vi "kSACommLVClient.vi"(1 "IP Address":string="localhost") -> ()   [LabVIEW 2019]
uses:
  C:/Users/tim/Documents/kSAComm LabView Sample/kSACommInterface.dll
  kSACommInterface.dll
  <vilib>/Platform/TimedLoop/XDataNode/timing_clust.ctl
  <vilib>/Platform/TimedLoop/XDataNode/nitl_modes.ctl
  <vilib>/Platform/TimedLoop/XDataNode/wakeup.ctl
  <vilib>/platform/TimedLoop/XDataNode/XDataNode.xnode
  <vilib>/regexp/Match Regular Expression.xnode
  <vilib>/Platform/TimedLoop/XDataNode/XDNodeRunTimeDep.lvlib
panel:
  out "Laser Command Response":string
  out "Register Data Items":bool
  in  "Laser On/Off":bool
  out "Connected":bool
  out "Exit App":bool
  out "Issue Text Command":bool
  in  "Tab Control":T1(tab)
  in  "Start/Stop Acquire":bool
  in  "Duration Type":i32(ring) items=["DURATION_TIME", "DURATION_DATA_POINTS", "DURATION_UNLIMITED"]
  in  "Run Name":string="LabVIEWTest"
  in  "Number of Samples":i16=1
  in  "Duration":dbl=60.0
  out "Array":cluster{"Id":u32, "Name":string}[](array[cluster])
  out "size(s)":i32
  out "Available Markers":u32
  in  "Show All Markers":bool
  in  "Marker":u32=1
  in  "Table Control":string[][](table)=[["0", "2", "Elapsed Time", " "], ["8", "0", "Data Point", ""], ["41059", "6", "Temperature", ""], ["41029", "6", "Curvature", ""]]
  in  "Data Frequency (ms)":i32=100 min=100 step=100
  out "Text Command Results":string
  in  "Send Text Command":bool
  in  "Command":string(combo)
  out "IssueCommand":i32(ring) items=["ERR_SUCCESS"=0, "ERR_CONNECTION"=-5, "ERR_STATE"=-4, "ERR_PARAM"=-3, "ERR_UNKOWN"=-2, "ERR_GENERAL"=-1]
  out "Last Error":string
  in  "OK Button":bool
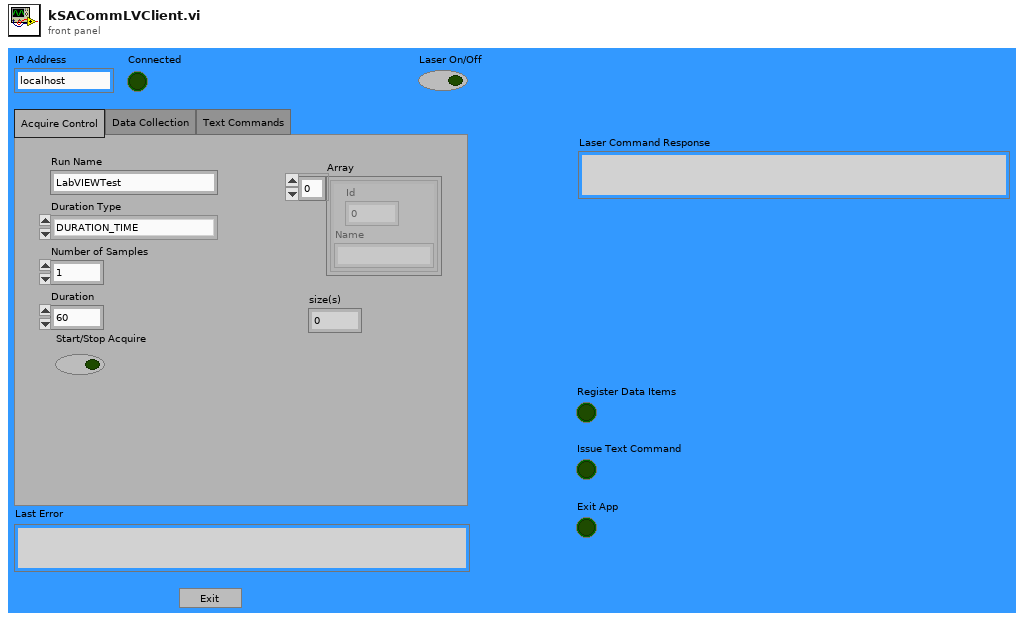
[diagram p1: front panel]
types:
  T1 = enum32{"Acquire Control", "Data Collection", "Text Commands"}
  T2 = typedef "XDNodeRunTimeDep.lvlib/timing_clust.ctl" = cluster{"Expected End [f-1]":u64, "Actual End [f-1]":u64, "Finished Late? [f-1]":bool, "Expected End [i-1]":u64, "Actual End [i-1]":u64, "Finished Late? [i-1]":bool, "Expected Start [i]":u64, "Actual Start [i]":u64, "Expected Start [f]":u64, "Actual Start [f]":u64, "Source Name":string, "Structure Name":string, "Period":i64, "Deadline":i64, "Offset":i64, "Start":i64, "Priority":i32, "Timeout":i32, "Mode":T3, "Wakeup Reason":T4, "Error":errorcluster, "Source Type":string, "Secondary Source Type":string, "Global End Time":u64, "Global Start Time":u64, "Frame Duration":u64, "Iteration Duration":u64, "Assigned CPU":i32, "I/O Scan Engine Mode":u32}
  T3 = typedef "XDNodeRunTimeDep.lvlib/nitl_modes.ctl" = enum32{"No Change", "Process missed periods, maintain original phase", "Discard missed periods, maintain original phase", "Process missed periods, ignore original phase", "Discard missed periods, ignore original phase"}
  T4 = typedef "XDNodeRunTimeDep.lvlib/wakeup.ctl" = enum32{"Normal", "Aborted", "Asynchronous wakeup", "Timing source error", "Timed loop error", "Timeout"}
  T5 = enum8{"Enabled", "Disabled", "Disabled and Grayed Out"}
  T6 = typedef "eventvkey.ctl" = enum16{"ASCII", "Enter", "Return", "Shift", "Ctrl", "Alt", "Cmd", "Opt", "Caps", "NumLock", "Clear", "Break", "Up", "Down", "Left", "Right", "Insert", "Delete", "Home", "End", "PageUp", "PageDown", "Escape", "Help", "Pause", "ScrollLock", "F1", "F2", "F3", "F4", "F5", "F6", "F7", "F8", "F9", "F10", "F11", "F12", "F13", "F14", "F15", "F16", "F17", "F18", "F19", "F20", "F21", "F22", "F23", "F24", "Play", "VolumeUp", "VolumeDown", "Mute", "Two Byte Char"}
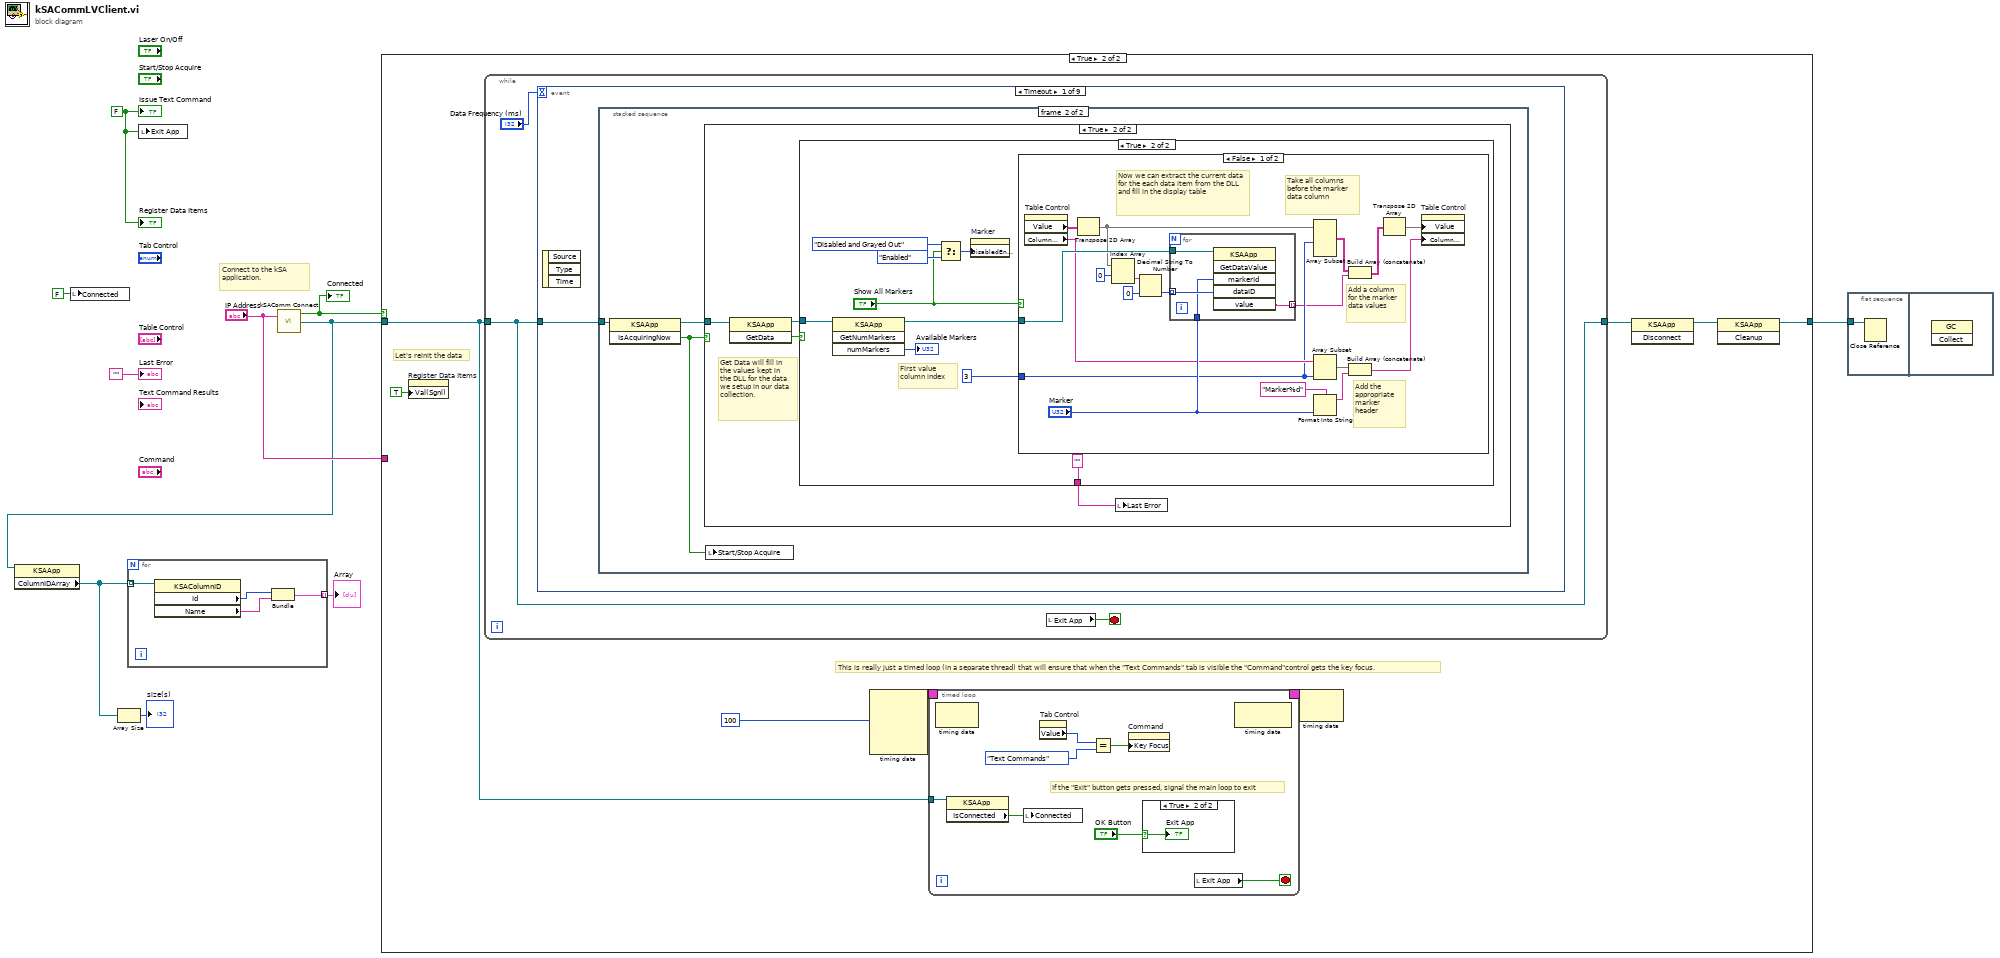
[diagram p0: block diagram]
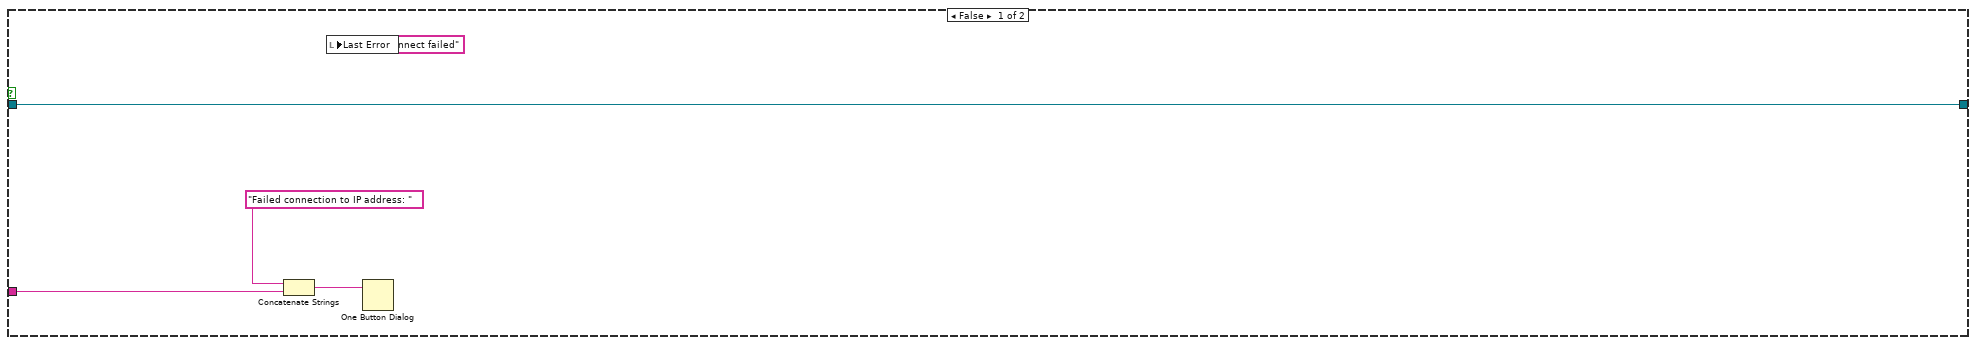
[diagram p2: hidden frame]
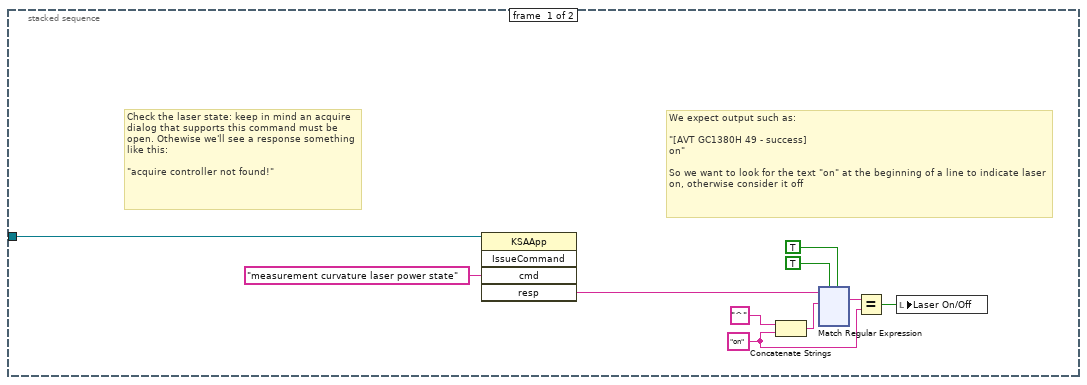
[diagram p4: hidden frame]
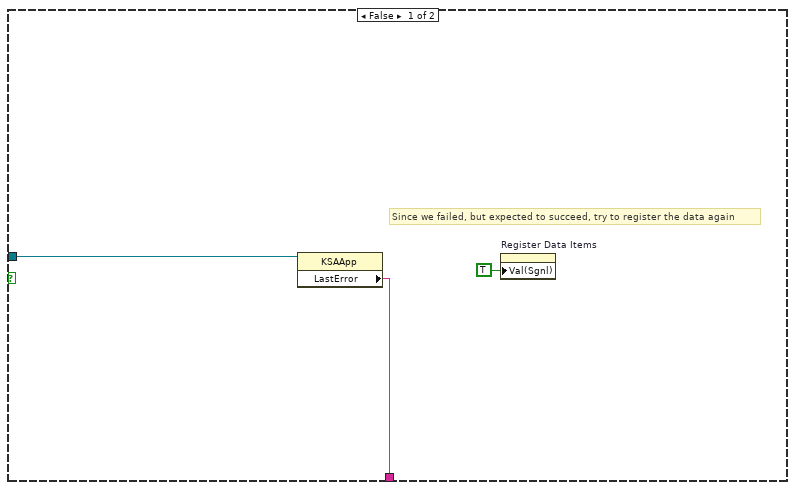
[diagram p6: hidden frame]
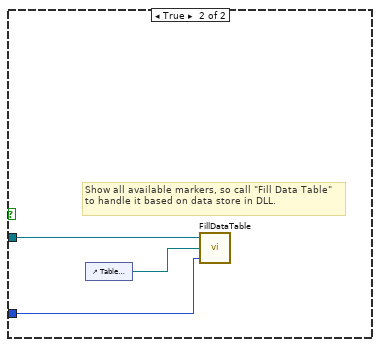
[diagram p7: hidden frame]
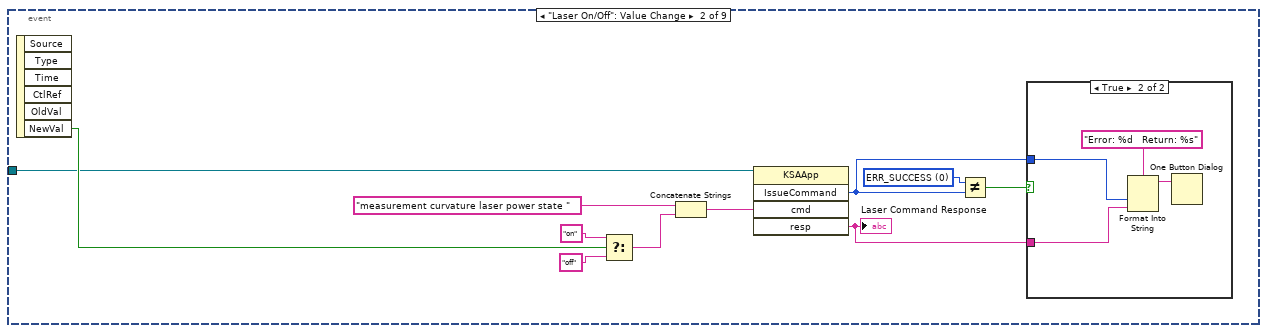
[diagram p8: hidden frame]
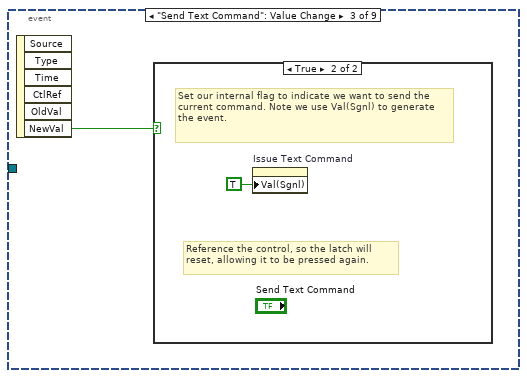
[diagram p10: hidden frame]
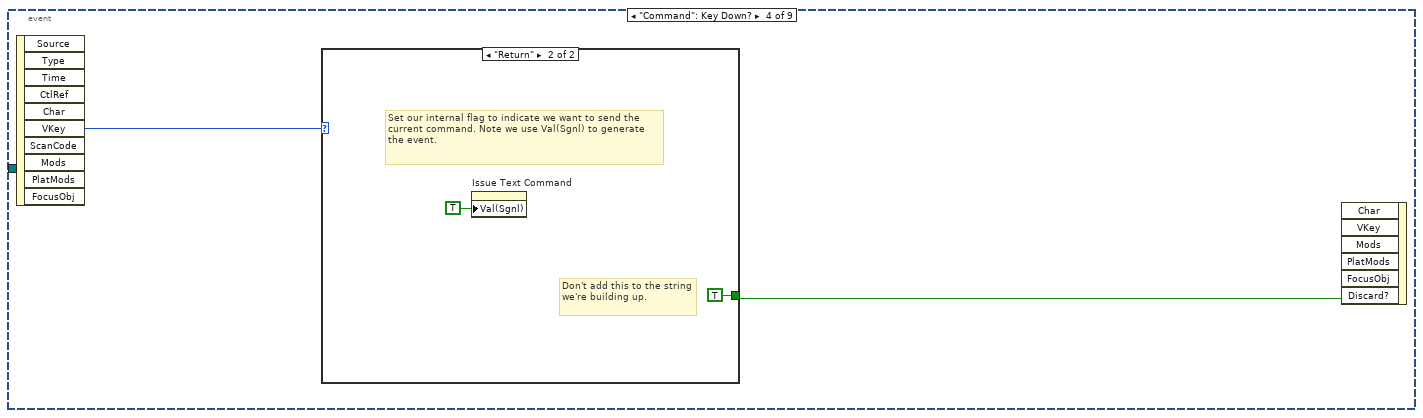
[diagram p12: hidden frame]
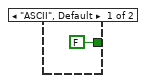
[diagram p13: hidden frame]
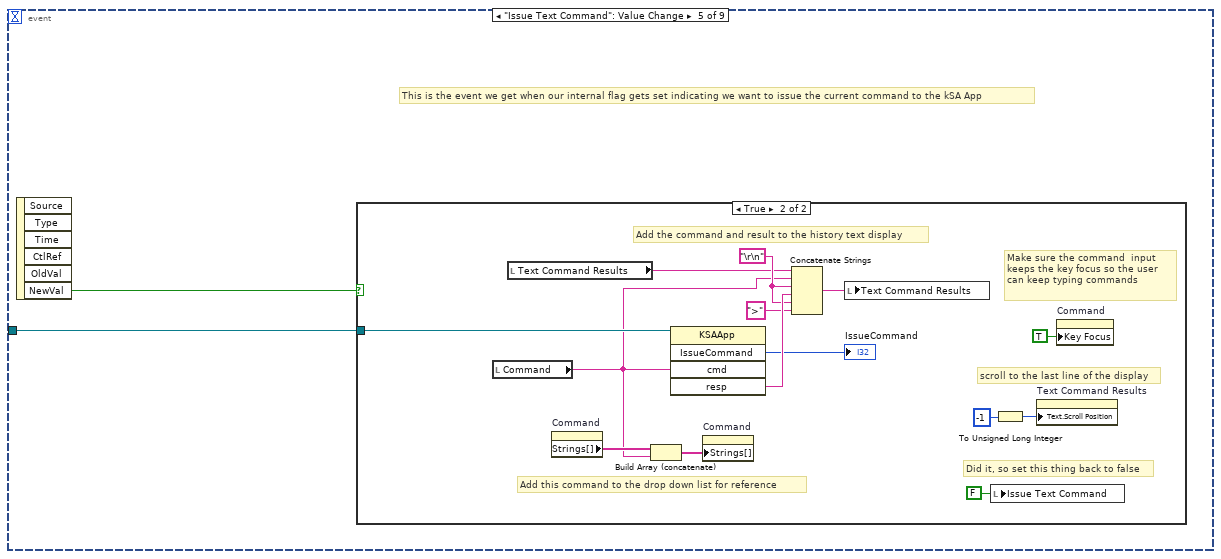
[diagram p14: hidden frame]
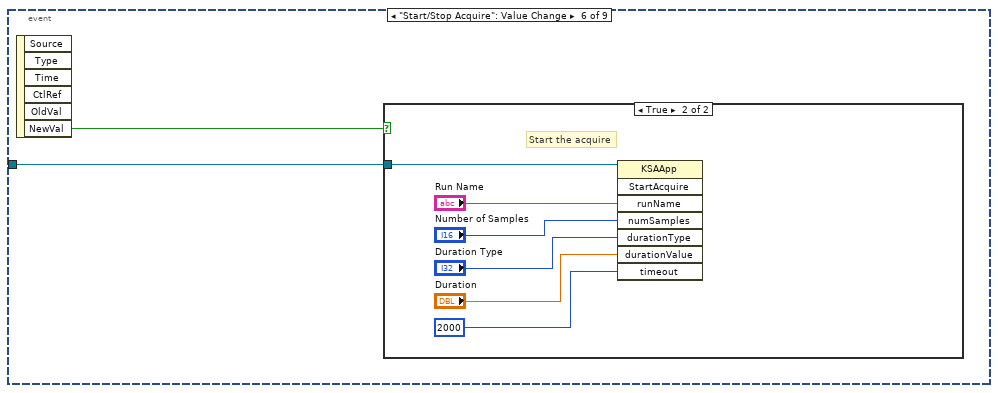
[diagram p16: hidden frame]
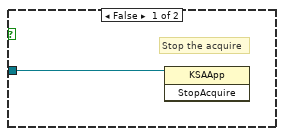
[diagram p17: hidden frame]
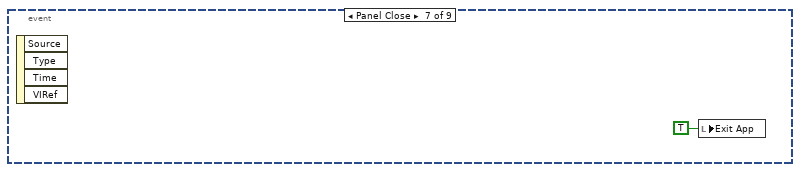
[diagram p18: hidden frame]
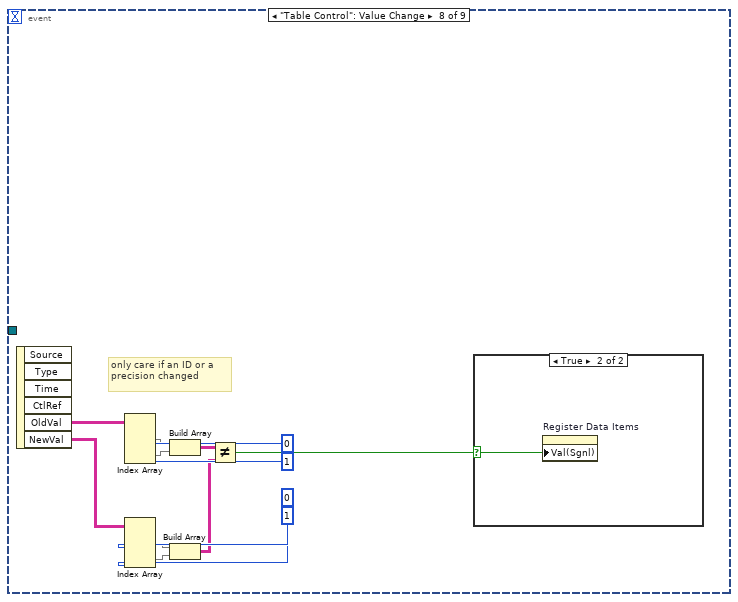
[diagram p19: hidden frame]
diagram:
  w8 = FALSE ("Send Text Command")
  # "Connect to the kSA application."
  n1 = local write "Connected"(FALSE ("Connected")) -> ()
  n2 = local write "Exit App"(w8) -> ()
  n3 = call "kSAComm Connect.vi"("IP Address"="IP Address") -> ("Connect"=w9:bool, "kSAComm ref out"=w4:refnum<k24>)  [unwired: 2 in]
  "Connected" <- w9
  n4 = property class="KSAApp"(reference=w4) -> ("ColumnIDArray"=w2:refnum<k24>[])  [unwired: 1 in, 2 out]
  n5 = Array Size(array=w2) -> (size(s)=→"size(s)":i32)
  n6 = for {
    tunnel: w2 -> [w14] mode=indexing
    tunnel: [w11] -> w3 mode=indexing
    n7 = property class="KSAColumnID"(reference=w14) -> ("Id"=w13:u32, "Name"=w12:string)  [unwired: 1 in, 2 out]
    n8 = Bundle("Id"=w13, "Name"=w12) -> (w11:cluster{"Id":u32, "Name":string})  [unwired: 1 in]
  }
  "Array" <- w3
  n9 = case shown="True" w9 {
    tunnel: w4 -> [w18 w23]
    tunnel: [w18 w21] -> w5
    tunnel: "IP Address" -> [w16 _]
    frame False {
      n10 = Concatenate Strings("Failed connection to IP address: ", w16) -> (w15:string)
      n11 = local write "Last Error"("Connect failed" ("Error")) -> ()
      n12 = One Button Dialog(message=w15) -> ()  [unwired: 1 in, 1 out]
    }
    frame True {
      # "This is really just a timed loop (in a separate thread) that will ensure that when the \"Text Commands\" tab is visible the \"Command\"control gets the key focus."
      # "Let's reinit the data"
      n13 = property on="Register Data Items" class="Bool (strict)"("Val(Sgnl)"=TRUE ("Value (Signaling)")) -> ()  [unwired: 2 in, 2 out]
      n14 = while {
        tunnel: w23 -> [w42]
        tunnel: [w42] -> w20
        stop <- w43 stop-if-true
        n15 = event shown="[0] Timeout" {
          selector: _ -> [_ _ _ _ _ _ _ _ _]
          dyn-events: _ -> [_ _ _ _ _ _ _ _ _]
          timeout: "Data Frequency (ms)" -> [_ _ _ _ _ _ _ _ _]
          tunnel: w42 -> [w45 w215 _ _ w236 w252 _ w263 w278]
          tunnel: [_ _ _ _ _ _ _ w263 _] -> _
          event Timeout {
            n16 = event-data() -> ()  [unwired: 1 in, 3 out]
            n17 = stacked-sequence {
              tunnel: w45 -> [w49 w170]
              frame #0 {
                w46 = "on" ("regular expression")
                # "Check the laser state: keep in mind an acquire dialog that supports this command must be open. Othewise we'll see a response something like this:\n\n\"acquire controller not found!\""
                # "We expect output such as:\n\n\"[AVT GC1380H 49 - success]\non\"\n\nSo we want to look for the text \"on\" at the beginning of a line to indicate laser on, otherwise consider it off"
                n18 = invoke class="KSAApp" method="IssueCommand"(reference=w49, "cmd"="measurement curvature laser power state") -> ("resp"=w55:string)  [unwired: 3 in, 4 out]
                n19 = Concatenate Strings("^", w46) -> (w47:string)
                n20 = xnode "Match Regular Expression"("input string"=w55, "regular expression"=w47, "ignore case? (F)"=TRUE, "multiline? (F)"=TRUE) -> ("whole match"=w52:string)  [unwired: 2 in, 4 out]
                n21 = Equal?(x=w52, y=w46) -> (x = y?=w50:bool)
                n22 = local write "Laser On/Off"(w50) -> ()
              }
              frame #1 {
                n23 = invoke class="KSAApp" method="IsAcquiringNow"(reference=w170) -> (reference out=w172:refnum<k24>, "IsAcquiringNow"=w171:bool)  [unwired: 2 in, 1 out]
                n24 = case shown="True" w171 {
                  tunnel: w172 -> [_ w176]
                  frame False {
                  }
                  frame True {
                    # "Get Data will fill in the values kept in the DLL for the data we setup in our data collection."
                    n25 = invoke class="KSAApp" method="GetData"(reference=w176) -> (reference out=w174:refnum<k24>, "GetData"=w175:bool)  [unwired: 2 in, 1 out]
                    n26 = case shown="True" w175 {
                      tunnel: w174 -> [w179 w181]
                      tunnel: [w178 "" ("LastError")] -> w173
                      frame False {
                        # "Since we failed, but expected to succeed, try to register the data again"
                        n27 = property class="KSAApp"(reference=w179) -> ("LastError"=w178:string)  [unwired: 1 in, 2 out]
                        n28 = property on="Register Data Items" class="Bool (strict)"("Val(Sgnl)"=TRUE ("Value (Signaling)")) -> ()  [unwired: 2 in, 2 out]
                      }
                      frame True {
                        # "First value column index"
                        n29 = invoke class="KSAApp" method="GetNumMarkers"(reference=w181) -> (reference out=w180:refnum<k24>, "numMarkers"=→"Available Markers":u32)  [unwired: 3 in, 2 out]
                        n30 = Select(t=T5."Disabled and Grayed Out" ("Disabled"), s="Show All Markers", f=T5."Enabled" ("Disabled")) -> (s? t:f=w186:T5)
                        n31 = property on="Marker" class="DigNum (strict)"("DisabledEnum"=w186) -> ()  [unwired: 2 in, 2 out]
                        n32 = case shown="False" "Show All Markers" {
                          tunnel: w180 -> [w206 w212]
                          tunnel: 3 ("First Data Column") -> [w193 w211]
                          frame False {
                            # "Add a column for the marker data values"
                            # "Take all columns before the marker data column"
                            # "Add the appropriate marker header"
                            # "Now we can extract the current data for the each data item from the DLL and fill in the display table"
                            n33 = property on="Table Control" class="Tbl (strict)"() -> ("Value"=w197:string[][], "Column Headers[]"=w196:string[])  [unwired: 2 in, 2 out]
                            n34 = Transpose 2D Array(2D array=w197) -> (transposed array=w194:string[][])
                            n35 = Index Array(array=w194, index (row)=0) -> (element=w203:string[])  [unwired: 1 in]
                            n36 = Decimal String To Number(string=w203, default (0L)=u32 0 ("default (0 I32)")) -> (number=w202:u32[])  [unwired: 1 in, 1 out]
                            n37 = for {
                              tunnel: w202 -> [w209] mode=indexing
                              tunnel: w206 -> [w210]
                              tunnel: [w208] -> w191 mode=indexing
                              tunnel: "Marker" -> [w207]
                              n38 = invoke class="KSAApp" method="GetDataValue"(reference=w210, "markerId"=w207, "dataID"=w209) -> ("value"=w208:string)  [unwired: 3 in, 5 out]
                            }
                            n39 = Array Subset(array=w194, length (row)=w193) -> (w192:string[][])  [unwired: 3 in]
                            n40 = Array Subset(array=w196, length=w193) -> (w198:string[])  [unwired: 1 in]
                            n41 = Format Into String(format string="Marker%d", "Marker") -> (resulting string=w199:string)  [unwired: 2 in, 1 out]
                            n42 = Build Array (concatenate)(w192, w191) -> (w190:string[][])
                            n43 = Build Array (concatenate)(w198, w199) -> (w189:string[])
                            n44 = Transpose 2D Array(2D array=w190) -> (transposed array=w195:string[][])
                            n45 = property on="Table Control" class="Tbl (strict)"("Value"=w195, "Column Headers[]"=w189) -> ()  [unwired: 2 in, 2 out]
                          }
                          frame True {
                            # "Show all available markers, so call \"Fill Data Table\" to handle it based on data store in DLL."
                            n46 = control-ref of="Table Control"() -> (w213:refnum<vi>)
                            n47 = call "FillDataTable.vi"("First Data Column Index"=w211, "Tbl Refnum"=w213, "kSAComm ref"=w212) -> ()  [unwired: 1 in]
                          }
                        }
                      }
                    }
                    n48 = local write "Last Error"(w173) -> ()
                  }
                }
                n49 = local write "Start/Stop Acquire"(w171) -> ()
              }
            }
          }
          event "Laser On/Off": Value Change {
            w216 = 0 items=["ERR_SUCCESS"=0, "ERR_CONNECTION"=-5, "ERR_STATE"=-4, "ERR_PARAM"=-3, "ERR_UNKOWN"=-2, "ERR_GENERAL"=-1] ("IssueCommand")
            n50 = event-data() -> ("NewVal"=w224:bool)  [unwired: 1 in, 5 out]
            n51 = Select(t="on", s=w224, f="off") -> (s? t:f=w220:string)
            n52 = Concatenate Strings("measurement curvature laser power state ", w220) -> (w219:string)
            n53 = invoke class="KSAApp" method="IssueCommand"(reference=w215, "cmd"=w219) -> ("IssueCommand"=w214:i32, "resp"=w217:string)  [unwired: 3 in, 3 out]
            "Laser Command Response" <- w217
            n54 = Not Equal?(x=w216, y=w214) -> (x != y?=w218:bool)
            n55 = case shown="True" w218 {
              tunnel: w217 -> [_ w227]
              tunnel: w214 -> [_ w228]
              frame False {
              }
              frame True {
                n56 = Format Into String(format string="Error: %d   Return: %s", w228, w227) -> (resulting string=w225:string)  [unwired: 2 in, 1 out]
                n57 = One Button Dialog(message=w225) -> ()  [unwired: 1 in, 1 out]
              }
            }
          }
          event "Send Text Command": Value Change {
            n58 = event-data() -> ("NewVal"=w229:bool)  [unwired: 1 in, 5 out]
            n59 = case shown="True" w229 {
              frame False {
              }
              frame True {
                # "Set our internal flag to indicate we want to send the current command. Note we use Val(Sgnl) to generate the event."
                # "Reference the control, so the latch will reset, allowing it to be pressed again."
                n60 = property on="Issue Text Command" class="Bool (strict)"("Val(Sgnl)"=TRUE) -> ()  [unwired: 2 in, 2 out]
              }
            }
          }
          event "Command": Key Down? {
            n61 = event-data() -> ("VKey"=w232:T6)  [unwired: 1 in, 9 out]
            n62 = case shown="\"Return\"" w232 {
              tunnel: [FALSE TRUE] -> w231
              frame "ASCII", Default {
              }
              frame "Return" {
                # "Don't add this to the string we're building up."
                # "Set our internal flag to indicate we want to send the current command. Note we use Val(Sgnl) to generate the event."
                n63 = property on="Issue Text Command" class="Bool (strict)"("Val(Sgnl)"=TRUE) -> ()  [unwired: 2 in, 2 out]
              }
            }
            n64 = event-data("Discard?"=w231) -> ()  [unwired: 6 in, 1 out]
          }
          event "Issue Text Command": Value Change {
            # "This is the event we get when our internal flag gets set indicating we want to issue the current command to the kSA App"
            n65 = event-data() -> ("NewVal"=w237:bool)  [unwired: 1 in, 5 out]
            n66 = case shown="True" w237 {
              tunnel: w236 -> [_ w246]
              frame False {
              }
              frame True {
                w244 = "\r\n"
                # "Make sure the command  input keeps the key focus so the user can keep typing commands"
                # "scroll to the last line of the display"
                # "Add the command and result to the history text display"
                # "Add this command to the drop down list for reference"
                # "Did it, so set this thing back to false"
                n67 = local read "Command"() -> (w241:string)
                n68 = local read "Text Command Results"() -> (w243:string)
                n69 = property on="Command" class="CmbBox"() -> ("Strings[]"=w242:string[])  [unwired: 2 in, 2 out]
                n70 = Build Array (concatenate)(w242, w241) -> (w240:string[])
                n71 = invoke class="KSAApp" method="IssueCommand"(reference=w246, "cmd"=w241) -> ("IssueCommand"=→"IssueCommand":i32, "resp"=w251:string)  [unwired: 3 in, 3 out]
                n72 = property on="Command" class="CmbBox"("Strings[]"=w240) -> ()  [unwired: 2 in, 2 out]
                n73 = Concatenate Strings(w243, w241, w244, w251, w244, ">" ("string")) -> (w250:string)
                n74 = local write "Text Command Results"(w250) -> ()
                n75 = local write "Issue Text Command"(FALSE ("Issue Text Command")) -> ()
                n76 = To Unsigned Long Integer(number=-1) -> (unsigned 32bit integer=w249:u32)
                n77 = property on="Text Command Results" class="Str"("Text.Scroll Position"=w249) -> ()  [unwired: 2 in, 2 out]
                n78 = property on="Command" class="CmbBox"("Key Focus"=TRUE) -> ()  [unwired: 2 in, 2 out]
              }
            }
          }
          event "Start/Stop Acquire": Value Change {
            n79 = event-data() -> ("NewVal"=w253:bool)  [unwired: 1 in, 5 out]
            n80 = case shown="True" w253 {
              tunnel: w252 -> [w254 w260]
              frame False {
                # "Stop the acquire"
                n81 = invoke class="KSAApp" method="StopAcquire"(reference=w254) -> ()  [unwired: 2 in, 3 out]
              }
              frame True {
                # "Start the acquire"
                n82 = invoke class="KSAApp" method="StartAcquire"(reference=w260, "runName"="Run Name", "numSamples"="Number of Samples", "durationType"="Duration Type", "durationValue"="Duration", "timeout"=2000) -> ()  [unwired: 2 in, 8 out]
              }
            }
          }
          event Panel Close {
            n83 = event-data() -> ()  [unwired: 1 in, 4 out]
            n84 = local write "Exit App"(TRUE ("Exit App")) -> ()
          }
          event "Table Control": Value Change {
            # "only care if an ID or a precision changed"
            n85 = event-data() -> ("OldVal"=w275:string[][], "NewVal"=w264:string[][])  [unwired: 1 in, 4 out]
            n86 = Index Array(array=w275, index (col) #1=0 ("disabled index (col)"), index (col) #2=1 ("index (col)")) -> (element #1=w270:string[], element #2=w269:string[])  [unwired: 2 in]
            n87 = Index Array(array=w264, index (col) #1=0 ("disabled index (col)"), index (col) #2=1 ("index (col)")) -> (element #1=w266:string[], element #2=w265:string[])  [unwired: 2 in]
            n88 = Build Array(w270, w269) -> (w268:string[][])
            n89 = Build Array(w266, w265) -> (w267:string[][])
            n90 = Not Equal?(x=w268, y=w267) -> (x != y?=w262:bool)
            n91 = case shown="True" w262 {
              selector: w262 -> [_ w276]
              frame False {
              }
              frame True {
                n92 = property on="Register Data Items" class="Bool (strict)"("Val(Sgnl)"=w276) -> ()  [unwired: 2 in, 2 out]
              }
            }
          }
          event "Register Data Items": Value Change {
            n93 = event-data() -> ("NewVal"=w277:bool)  [unwired: 1 in, 5 out]
            n94 = case shown="True" w277 {
              tunnel: w278 -> [_ w285]
              frame False {
              }
              frame True {
                # "Name Column"
                # "Precision Column"
                # "Data ID Column"
                # "Make sure it's a valid reference. If there's less than 2 rows in the data table, for some reason, it goes null."
                # "We did it, so reset out internal flag"
                # "Whenever we have a change in the set of data we want to collect, we need to clear out the current set, register each item, then call SetData to let the kSA app know about the change."
                n95 = local read "Table Control"() -> (w282:string[][])
                n96 = invoke class="KSAApp" method="ClearDataCollection"(reference=w285) -> (reference out=w284:refnum<k24>)  [unwired: 2 in, 2 out]
                n97 = Index Array(array=w282, index (col) #1=0 ("disabled index (col)"), index (col) #2=1 ("index (col)"), index (col) #3=2 ("index (col)")) -> (element #1=w291:string[], element #2=w294:string[], element #3=w293:string[])  [unwired: 3 in]
                n98 = Decimal String To Number(string=w291, default (0L)=u32 0 ("default (0 I32)")) -> (number=w290:u32[])  [unwired: 1 in, 1 out]
                n99 = Decimal String To Number(string=w294) -> (number=w292:i32[])  [unwired: 2 in, 1 out]
                n100 = for {
                  tunnel: w293 -> [w304] mode=indexing
                  tunnel: w292 -> [w303] mode=indexing
                  tunnel: w284 -> [w302]
                  tunnel: [w301] -> w279
                  tunnel: w290 -> [w300] mode=indexing
                  n101 = invoke class="KSAApp" method="RegisterDataItem"(reference=w302, "name"=w304, "id"=w300, "precision"=w303) -> (reference out=w301:refnum<k24>)  [unwired: 2 in, 5 out]
                }
                n102 = Not Equal?(x=w279, y=refnum<k24> refnum ("reference out")) -> (x != y?=w281:bool)
                n103 = case shown="True" w281 {
                  tunnel: w279 -> [_ w297]
                  frame False {
                  }
                  frame True {
                    n104 = invoke class="KSAApp" method="SetData"(reference=w297) -> (reference out=w295:refnum<k24>, "SetData"=w296:bool)  [unwired: 2 in, 1 out]
                    n105 = case shown="False" w296 {
                      tunnel: w295 -> [w298 _]
                      frame False {
                        n106 = property class="KSAApp"(reference=w298) -> ("LastError"=w299:string)  [unwired: 1 in, 2 out]
                        n107 = local write "Last Error"(w299) -> ()
                      }
                      frame True {
                      }
                    }
                  }
                }
                n108 = local write "Register Data Items"(FALSE ("Register Data Items")) -> ()
              }
            }
          }
        }
        n109 = local read "Exit App"() -> (w43:bool)
      }
      n110 = node-c288(i64 100 ("Period")) -> (w26:T2)  [unwired: 3 in]
      n111 = timed-loop {
        timing: w26 -> [_]
        timing-out: [_] -> w25
        tunnel: w23 -> [w30]
        stop <- w31 stop-if-true
        # "If the \"Exit\" button gets pressed, signal the main loop to exit"
        n112 = node-c288() -> ()  [unwired: 1 in, 1 out]
        n113 = property class="KSAApp"(reference=w30) -> ("IsConnected"=w28:bool)  [unwired: 1 in, 2 out]
        n114 = local write "Connected"(w28) -> ()
        n115 = property on="Tab Control" class="TabCtl (strict)"() -> ("Value"=w33:T1)  [unwired: 2 in, 2 out]
        n116 = Equal?(x=w33, y=T1."Text Commands") -> (x = y?=w32:bool)
        n117 = property on="Command" class="CmbBox"("Key Focus"=w32) -> ()  [unwired: 2 in, 2 out]
        n118 = case shown="True" "OK Button" {
          selector: "OK Button" -> [_ w35]
          frame False {
          }
          frame True {
            "Exit App" <- w35
          }
        }
        n119 = local read "Exit App"() -> (w31:bool)
        n120 = node-c288() -> ()  [unwired: 1 in, 1 out]
      }
      n121 = node-c288(w25) -> ()  [unwired: 1 out]
      n122 = invoke class="KSAApp" method="Disconnect"(reference=w20) -> (reference out=w22:refnum<k24>)  [unwired: 2 in, 2 out]
      n123 = invoke class="KSAApp" method="Cleanup"(reference=w22) -> (reference out=w21:refnum<k24>)  [unwired: 2 in, 2 out]
    }
  }
  n124 = flat-sequence {
    tunnel: w5 -> [w305]
    frame #0 {
      n125 = Close Reference(reference=w305) -> ()  [unwired: 1 in, 1 out]
    }
    frame #1 {
      n126 = invoke class="GC" method="Collect"() -> ()  [unwired: 3 in, 3 out]
    }
  }
  "Last Error" <- "" ("Error")
  "Issue Text Command" <- w8
  "Register Data Items" <- w8
